vi "Addressing_sendSingleCMD.vi"(6 "address_group":u16, 7 "device_handle":i32, 8 "error in (no error)":errorcluster, 9 "DATA":u32, 10 "Command":T1="SEARCHADDRH", 11 "addressing_type":T2) -> (0 "error out":errorcluster, 3 "Answer Received?":bool)   [LabVIEW 2014, in "Driver_interaction.lvlib" / "Dali_usb_tridonics.lvclass"]
uses:
  Dali_usb_tridonics.lvclass
  Vendor/Controls/Addressing_type.ctl
  Controls/Commands enum.ctl
  Vendor/Dali_usb.lvlib
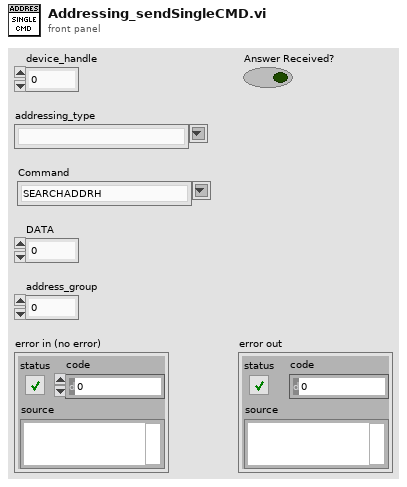
[diagram p1: front panel]
types:
  T1 = typedef "Driver_interaction.lvlib/Dali_usb_tridonics.lvclass/Commands enum.ctl" = string
  T2 = typedef "Dali_usb.lvlib/Addressing_type.ctl" = string
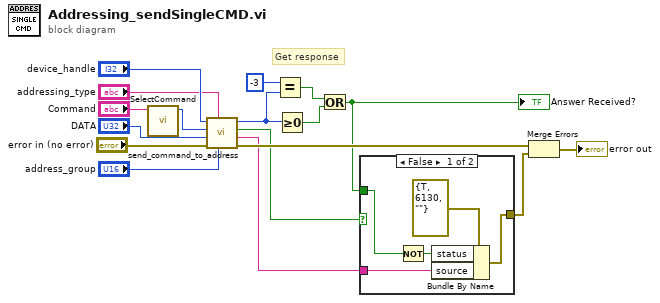
[diagram p0: block diagram]
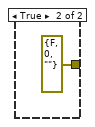
[diagram p2: hidden frame]
diagram:
  # "Get response"
  n1 = call "SelectCommand.vi"("Select Command"="Command") -> ("Command"=w8:u32)  [unwired: 10 in]
  n2 = call "send_command_to_address.vi"("address_group"="address_group", "addressing_type"="addressing_type", "error in (no error)"="error in (no error)", "command_data"="DATA", "command"=w8, "device_handle"="device_handle") -> ("error out"=w15:errorcluster, "failstring"=w12:string, "ok"=w11:bool, "response_command"=w3:i32)  [unwired: 2 in]
  n3 = Equal?(x=-3, y=w3) -> (x = y?=w4:bool)
  n4 = Greater Or Equal To 0?(x=w3) -> (x >= 0?=w5:bool)
  n5 = Or(x=w4, y=w5) -> (x .or. y?=w1:bool)
  "Answer Received?" <- w1
  n6 = case shown="False" w11 {
    tunnel: w12 -> [w21 _]
    tunnel: [w20 errorcluster {"status"=FALSE, "code"=0, "source"=""} ("error out")] -> w14
    tunnel: w1 -> [w19 _]
    frame False {
      n7 = Not(x=w19) -> (.not. x?=w18:bool)
      n8 = Bundle By Name(cluster=errorcluster {"status"=TRUE, "code"=6130, "source"=""} ("error out"), "status"=w18, "source"=w21) -> (w20:errorcluster)
    }
    frame True {
    }
  }
  n9 = Merge Errors(w15, w14) -> (→"error out":errorcluster)
